vi "HandelPickEvent.vi"(1 "Pick Settings":T1 {"Threshold" format="%.2f"}, 2 "gauss fit":bool) -> (0 "error out":errorcluster)   [LabVIEW 2009]
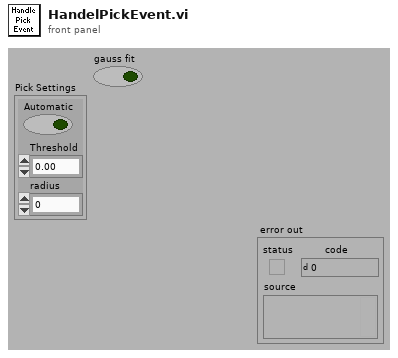
[diagram p1: front panel]
types:
  T1 = cluster{"Automatic":bool, "Threshold":dbl, "radius":i32}
  T2 = typedef "PickImage.ctl" = cluster{"Rawdata":T3, "Mask":T3, "Display":T3, "Coefficients (2D)":sgl[][], "Destroy Index":u32}
  T3 = typedef "IMAQ Image.ctl" = refnum<image>
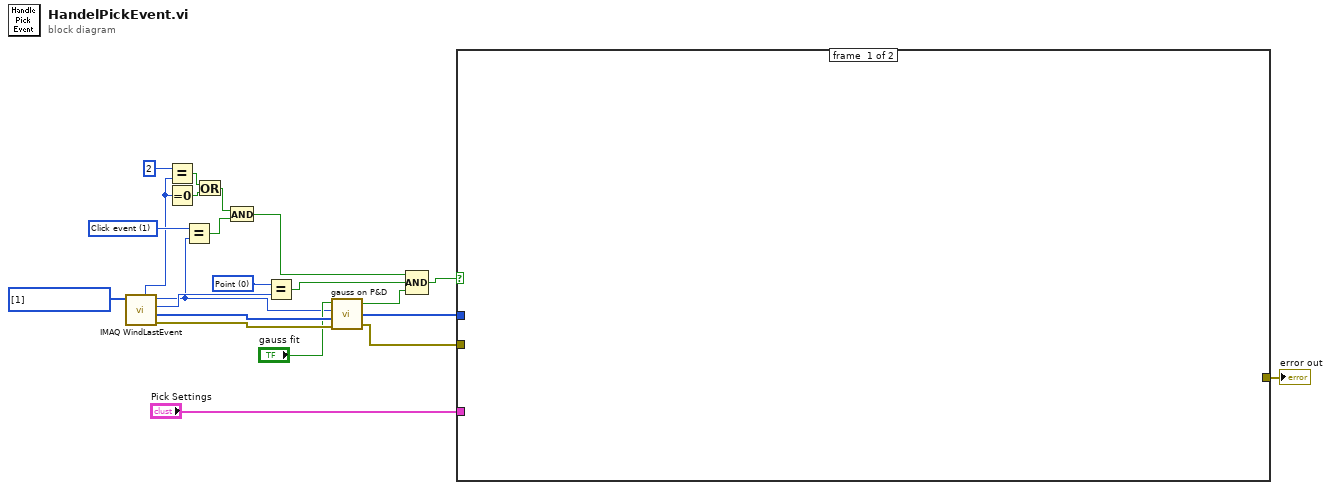
[diagram p0: block diagram]
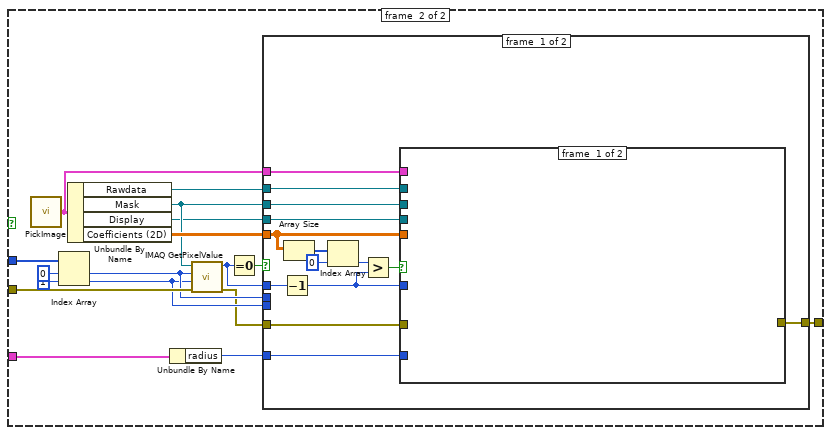
[diagram p2: hidden frame]
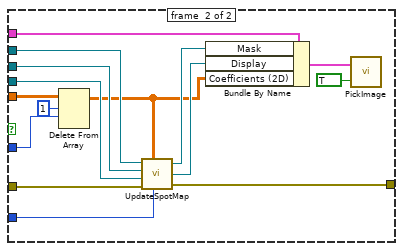
[diagram p3: hidden frame]
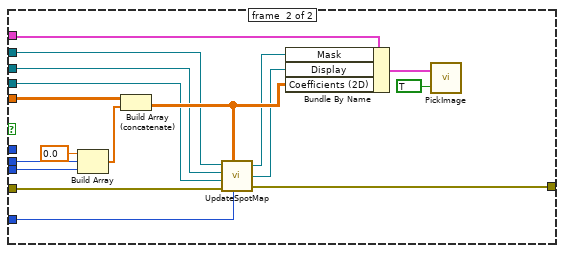
[diagram p4: hidden frame]
diagram:
  w16 = 0 items=["Point", "Line", "Rectangle", "Oval", "Polygon", "Free", "Annulus", "Rotated Rectangle", "Zoom", "Pan", "MultiLine", "FreeLine"] ("Tool")
  w19 = i32[] [1] items=["No  event", "Click event", "Draw event", "Move event", "Size event", "Scroll event", "Activate event", "Close event", "Double click event"] ("Events list (all)")
  w20 = 1 items=["No  event", "Click event", "Draw event", "Move event", "Size event", "Scroll event", "Activate event", "Close event", "Double click event"] ("Event")
  n1 = call "IMAQ WindLastEvent"("Events list (all)"=w19) -> ("error out"=w4:errorcluster, "Coordinates"=w10:i32[], "Tool"=w17:i32, "Event"=w1:i32, "Window Number (0...15)"=w13:i32)  [unwired: 5 in, 1 out]
  n2 = Equal?(x=2, y=w13) -> (x = y?=w12:bool)
  n3 = Equal To 0?(x=w13) -> (x = 0?=w14:bool)
  n4 = Equal?(x=w20, y=w1) -> (x = y?=w21:bool)
  n5 = Or(x=w12, y=w14) -> (x .or. y?=w15:bool)
  n6 = And(x=w15, y=w21) -> (x .and. y?=w8:bool)
  n7 = Equal?(x=w16, y=w17) -> (x = y?=w7:bool)
  n8 = call "gauss on P&D.vi"("error in (no error)"=w4, "Coordinates"=w10, "click event"=w1, "gauss fit"="gauss fit") -> ("error out"=w3:errorcluster, "fitted \ncoordinates"=w9:i32[], "Fit successful"=w6:bool)
  n9 = Compound Arithmetic op=AND(w8, w7, w6) -> (w5:bool)
  n10 = case shown="True" w5 {
    tunnel: w9 -> [_ w39]
    tunnel: w3 -> [_ w36]
    tunnel: "Pick Settings" -> [_ w24]
    tunnel: [_ w23] -> w18
    frame #0 {
    }
    frame #1 {
      n11 = call "PickImage.vi"() -> ("Image (output)"=w31:T2)  [unwired: 2 in]
      n12 = Index Array(array=w39, index #1=0 ("index"), index #2=1 ("index")) -> (element #1=w33:i32, element #2=w32:i32)
      n13 = Unbundle By Name(w31) -> ("Rawdata"=w28:T3, "Mask"=w30:T3, "Display"=w27:T3, "Coefficients (2D)"=w34:sgl[][])
      n14 = Unbundle By Name(w24) -> ("radius"=w25:i32)
      n15 = call "IMAQ GetPixelValue"("Image"=w30, "X Coordinate"=w33, "Y Coordinate"=w32, "error in (no error)"=w36) -> ("Pixel Value (U8)"=w26:u8, "error out"=w29:errorcluster)  [unwired: 3 in, 2 out]
      n16 = Equal To 0?(x=w26) -> (x = 0?=w35:bool)
      n17 = case shown="True" w35 {
        tunnel: w34 -> [w49 w85]
        tunnel: w33 -> [_ w82]
        tunnel: w32 -> [_ w81]
        tunnel: w31 -> [w47 w79]
        tunnel: w30 -> [w45 w75]
        tunnel: w29 -> [w43 w73]
        tunnel: w28 -> [w46 w76]
        tunnel: w27 -> [w44 w74]
        tunnel: w26 -> [w48 _]
        tunnel: w25 -> [w41 w70]
        tunnel: [w40 w69] -> w23
        frame #0 {
          n18 = Decrement(x=w48) -> (x-1=w42:u8)
          n19 = Array Size(array=w49) -> (size(s)=w53:i32[])
          n20 = Index Array(array=w53, index=0) -> (element=w51:i32)
          n21 = Greater?(x=w51, y=w42) -> (0:w50:bool)
          n22 = case shown="True" w50 {
            tunnel: w49 -> [_ w68]
            tunnel: w42 -> [_ w66]
            tunnel: w47 -> [_ w61]
            tunnel: w46 -> [_ w60]
            tunnel: w45 -> [_ w59]
            tunnel: w44 -> [_ w58]
            tunnel: w43 -> [_ w57]
            tunnel: w41 -> [_ w55]
            tunnel: [_ w54] -> w40
            frame #0 {
            }
            frame #1 {
              n23 = Delete From Array(array=w68, length=1, index (row)=w66) -> (array with subset deleted=w56:sgl[][])  [unwired: 1 in, 1 out]
              n24 = call "UpdateSpotMap.vi"("Rawdata"=w60, "Coefficients"=w56, "Mask (input)"=w59, "Display Input"=w58, "radius"=w55, "error in (no error)"=w57) -> ("Mask (output)"=w63:T3, "Display (output"=w62:T3, "error out"=w54:errorcluster)
              n25 = Bundle By Name(cluster=w61, "Mask"=w63, "Display"=w62, "Coefficients (2D)"=w56) -> (w65:T2)
              n26 = call "PickImage.vi"("Get/Set"=TRUE, "Images (input)"=w65) -> ()  [unwired: 1 out]
            }
          }
        }
        frame #1 {
          n27 = Build Array(0.0 ("array"), w82, w81) -> (w84:dbl[])
          n28 = Build Array (concatenate) "Build Array"(w85, w84) -> (w77:dbl[][])
          n29 = call "UpdateSpotMap.vi"("Rawdata"=w76, "Coefficients"=w77, "Mask (input)"=w75, "Display Input"=w74, "radius"=w70, "error in (no error)"=w73) -> ("Mask (output)"=w72:T3, "Display (output"=w71:T3, "error out"=w69:errorcluster)
          n30 = Bundle By Name(cluster=w79, "Mask"=w72, "Display"=w71, "Coefficients (2D)"=w77) -> (w80:T2)
          n31 = call "PickImage.vi"("Get/Set"=TRUE, "Images (input)"=w80) -> ()  [unwired: 1 out]
        }
      }
    }
  }
  "error out" <- w18
